vi "GlobalRegEd px_triggerEN.vi"(4 "Pixel number":u8 max=99 step=1, 5 "Global Reg (default)":u32[](array[numeric])=[68228136, 235671609, 0, 0, 0, 0] format="%.0x") -> (1 "Global Regster (U32)":u32[](array[numeric]) format="%08x")   [LabVIEW 2015, in "VIPM2.lvlib"]
doc: "On a default Global Register value, enables only the trigger of the given pixel."
uses:
  VIPM2.lvlib
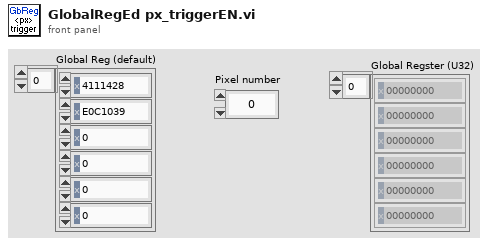
[diagram p1: front panel]
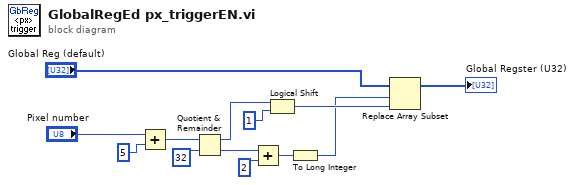
[diagram p0: block diagram]
diagram:
  n1 = Add(x="Pixel number", y=u8 5) -> (x+y=w11:u8)
  n2 = Quotient & Remainder(x=w11, y=u8 32) -> (x-y*floor(x/y)=w6:u8, floor(x/y)=w9:u8)
  n3 = Add(x=w9, y=u8 2) -> (x+y=w3:u8)
  n4 = Logical Shift(y=w6, x=u32 1) -> (x << y=w4:u32)
  n5 = To Long Integer(number=w3) -> (32bit integer=w2:i32)
  n6 = Replace Array Subset "Replace Array Subset"(array="Global Reg (default)", new element=w4, index=w2) -> (→"Global Regster (U32)":u32[])
